vi "Autosalvamento_adq.vi"() -> (0 "Quantidade de\narquivos adquiridos":i64, 3 "path":path)   [LabVIEW 2019]
panel:
  out "Horas":string
  out "Data":string
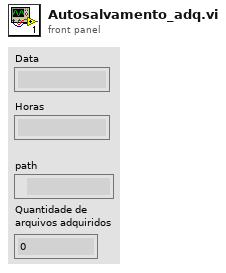
[diagram p1: front panel]
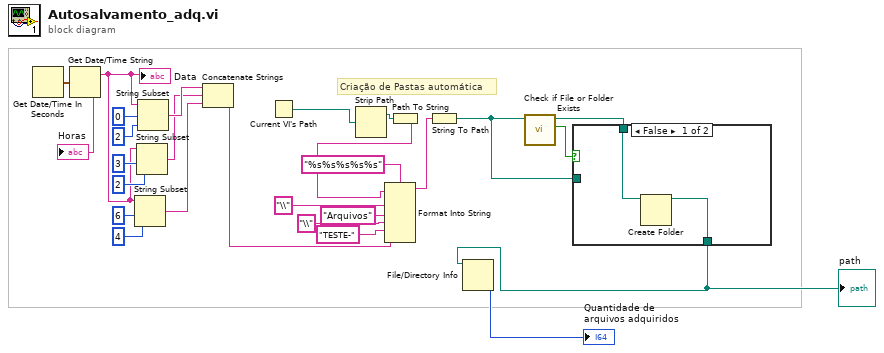
[diagram p0: block diagram]
diagram:
  # "Criação de Pastas automática"
  n1 = Get Date/Time In Seconds() -> (seconds since 1Jan1904=w27:timestamp)
  n2 = Get Date/Time String(seconds (now)=w27) -> (date string=w13:string, time string=→"Horas":string)  [unwired: 2 in]
  "Data" <- w13
  n3 = String Subset(string=w13, offset (0)=6, length (rest)=4 ("length (rest)")) -> (substring=w14:string)
  n4 = String Subset(string=w13, offset (0)=3, length (rest)=2 ("length (rest)")) -> (substring=w15:string)
  n5 = String Subset(string=w13, offset (0)=0, length (rest)=2 ("length (rest)")) -> (substring=w16:string)
  n6 = Concatenate Strings(w16, w15, w14) -> (w5:string)
  n7 = Current VI's Path() -> (path=w8:path)
  n8 = Strip Path(path=w8) -> (stripped path=w7:path)  [unwired: 1 out]
  n9 = Path To String(path=w7) -> (string=w6:string)
  n10 = Format Into String(format string="%s%s%s%s%s", initial string=w6, "\\" ("input 1"), "Arquivos" ("input 2"), "\\" ("input 1"), "TESTE-" ("input 2"), w5) -> (resulting string=w23:string)  [unwired: 1 in, 1 out]
  n11 = String To Path(string=w23) -> (path=w11:path)
  n12 = call <vilib>:"Check if File or Folder Exists.vi"("path"=w11) -> ("file or folder exists?"=w25:bool, "dup path"=w12:path)  [unwired: 8 in, 1 out]
  n13 = case shown="False" w25 {
    tunnel: w12 -> [w29 _]
    tunnel: [w28 w30] -> w9
    tunnel: w11 -> [_ w30]
    frame False {
      n14 = Create Folder(path (use dialog)=w29) -> (created path=w28:path)  [unwired: 2 in, 2 out]
    }
    frame True {
    }
  }
  "path" <- w9
  n15 = File/Directory Info(path=w9) -> (size=→"Quantidade de\narquivos adquiridos":i64)  [unwired: 1 in, 6 out]
